vi "All Child Values.vi"(11 "User in":refnum<class "User.lvclass">) -> (2 "All Values":refnum<class "Type.lvclass">[](array[class]))   [LabVIEW 2022 SP3, in "Test.lvlib" / "User.lvclass"]
uses:
  User.lvclass
  <vilib>/IlluminatedG/IG Conditum/Conditum/Columns/Type/Type.lvclass
  User.lvclass/User.ctl
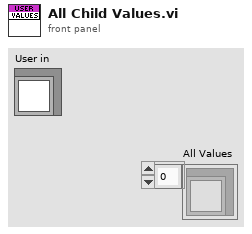
[diagram p1: front panel]
types:
  T1 = typedef "Test.lvlib/User.lvclass/Columns.ctl" = cluster{"Username":refnum<class "String.lvclass">, "Password":refnum<class "String.lvclass">, "Joined":refnum<class "Timestamp.lvclass">, "Last Activity":refnum<class "Timestamp.lvclass">, "Activated":refnum<class "Boolean.lvclass">, "Email":refnum<class "String.lvclass">, "Score":refnum<class "Integer.lvclass">}
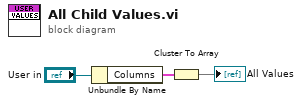
[diagram p0: block diagram]
diagram:
  n1 = Unbundle By Name("User in") -> ("Columns"=w2:T1)
  n2 = Cluster To Array(cluster=w2) -> (array=→"All Values":refnum<class "Type.lvclass">[])
